vi "MTS_AutoLaserPower.vi"(11 "Laser Color":enum16{"Blue", "Green", "Red"}(ring)) -> (0 "Error ?":bool, 1 "Laser 2 Position":dbl, 2 "Laser 1 Position":dbl, 3 "New Positions":u8[](array[numeric]))   [LabVIEW 2011]
panel:
  out "Progress":u8(slide) scale=0.0..100.0
  out "Laser Power":cluster{dbl[], dbl[]}(graph)
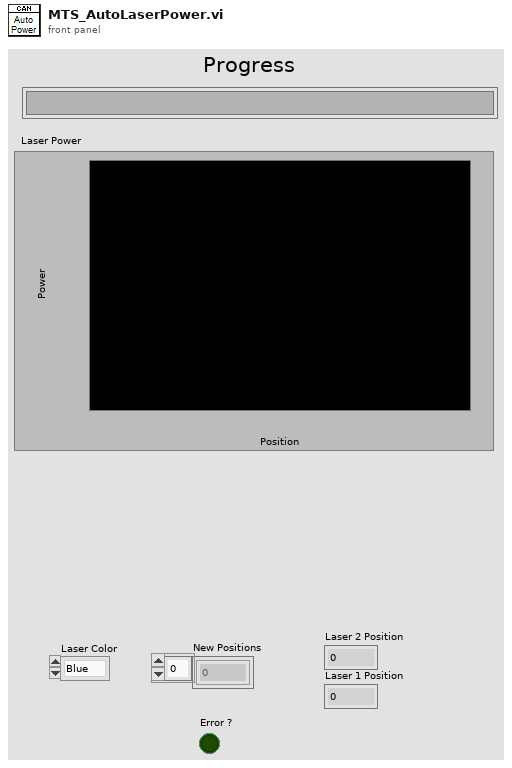
[diagram p1: front panel]
types:
  T1 = enum8{"STD, NO RTR", "STD,RTR", "XTD, NO RTR", "XTD, RTR"}
  T2 = cluster{"x":u32, "MSG type":enum8{"STD, NO RTR", "STD,RTR", "XTD, NO RTR", "XTD, RTR"}, "LEN 3":u8, u8[]}
  T3 = cluster{"x":u32, "MSG type":enum8{"STD, NO RTR", "STD,RTR", "XTD, NO RTR", "XTD, RTR"}, "LEN 3":u8, "Array":u8[]}
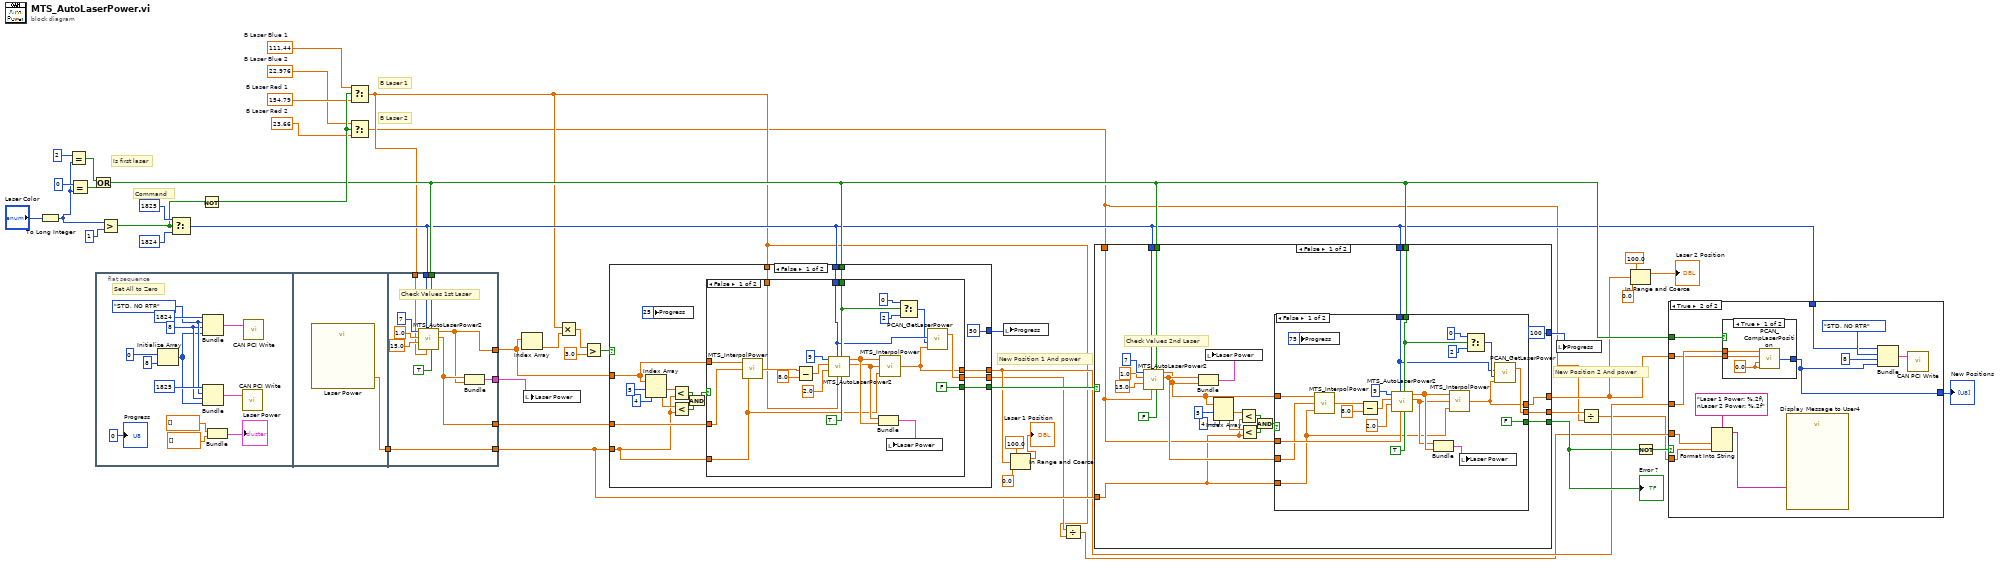
[diagram p0: block diagram]
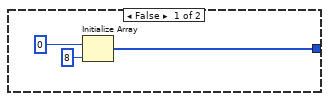
[diagram p2: hidden frame]
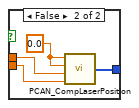
[diagram p3: hidden frame]
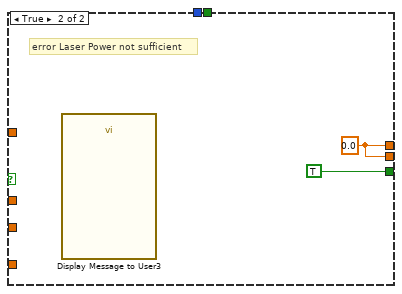
[diagram p4: hidden frame]
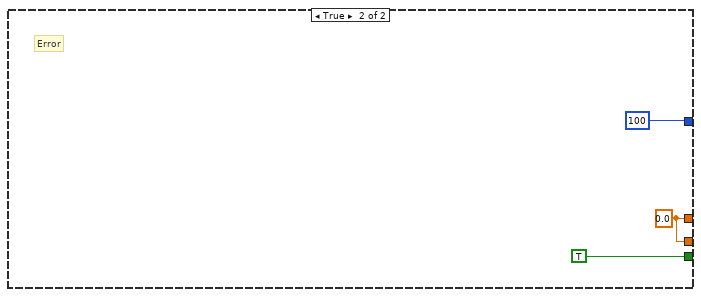
[diagram p5: hidden frame]
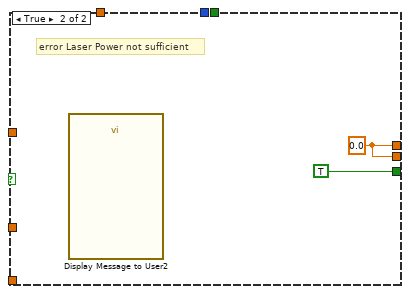
[diagram p6: hidden frame]
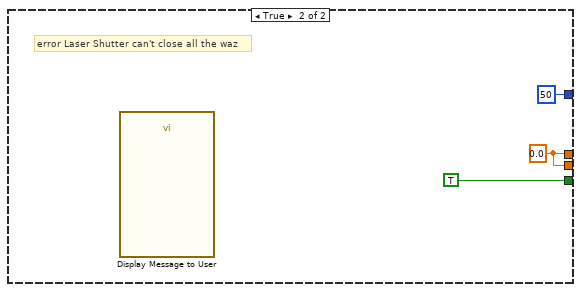
[diagram p7: hidden frame]
diagram:
  w28 = 23.66  # B Laser Red 2
  w30 = 154.79  # B Laser Red 1
  w29 = 22.976  # B Laser Blue 2
  w33 = 111.44  # B Laser Blue 1
  # "New Position 2 And power"
  # "New Position 1 And power"
  # "B Laser 2"
  # "B Laser 1"
  # "Is first laser"
  # "Command"
  n1 = To Long Integer(number="Laser Color") -> (32bit integer=w41:i32)
  n2 = Equal?(x=2, y=w41) -> (x = y?=w38:bool)
  n3 = Equal?(x=0, y=w41) -> (x = y?=w39:bool)
  n4 = Or(x=w38, y=w39) -> (x .or. y?=w21:bool)
  n5 = flat-sequence {
    tunnel: [w60] -> w37
    tunnel: w12 -> [w69]
    tunnel: w21 -> [w70]
    tunnel: [w63] -> w34
    tunnel: [w71] -> w25
    tunnel: w37 -> [w71]
    tunnel: [w64] -> w27
    tunnel: [w62] -> w9
    tunnel: w4 -> [w61]
    frame #0 {
      w54 = T1."STD, NO RTR" ("MSG type")
      w53 = u8 8 ("LEN 3")
      # "Set All to Zero"
      n6 = Initialize Array(u8 0, 8 ("dimension size")) -> (w52:u8[])
      n7 = Bundle("x"=u32 1824, "MSG type"=w54, "LEN 3"=w53, w52) -> (w57:T2)  [unwired: 1 in]
      n8 = Bundle("x"=u32 1825, "MSG type"=w54, "LEN 3"=w53, w52) -> (w51:T2)  [unwired: 1 in]
      n9 = Bundle(dbl[] [], dbl[] []) -> (→"Laser Power":cluster{dbl[], dbl[]})  [unwired: 1 in]
      n10 = call "CAN PCI Write.vi"("CAN_Message"=w51) -> ()  [unwired: 2 in, 1 out]
      n11 = call "CAN PCI Write.vi"("CAN_Message"=w57) -> ()  [unwired: 2 in, 1 out]
      "Progress" <- u8 0 ("Slide")
    }
    frame #1 {
      n12 = call "Laser Power"() -> ("Power ( µW )"=w60:dbl)  [unwired: 17 in, 2 out]
    }
    frame #2 {
      # "Check Values 1st Laser"
      n13 = call "MTS_AutoLaserPower2.vi"("Laser 1/3 ?"=TRUE, "Laser 1-2 ?"=w70, "Laser Power Callib"=w61, "CAN Adress"=w69, "Step"=15.0, "Offset"=1.0, "N Points"=7) -> ("Positions"=w64:dbl[], "Intensitys"=w63:dbl[])  [unwired: 2 in, 1 out]
      n14 = Bundle("Positions"=w64, "Intensitys"=w63) -> (w62:cluster{"Positions":dbl[], "Intensitys":dbl[]})  [unwired: 1 in]
    }
  }
  n15 = Greater?(x=w41, y=1) -> (0:w32:bool)
  n16 = Select(t=u32 1825 ("x"), s=w32, f=u32 1824 ("x")) -> (s? t:f=w12:u32)
  n17 = Not(x=w32) -> (.not. x?=w31:bool)
  n18 = Select(t=w33, s=w31, f=w30) -> (s? t:f=w4:dbl)
  n19 = Select(t=w29, s=w31, f=w28) -> (s? t:f=w1:dbl)
  n20 = Index Array(array=w34) -> (element=w8:dbl)  [unwired: 1 in]
  n21 = local write "Laser Power"(w9) -> ()
  n22 = Multiply(x=w4, y=w8) -> (x*y=w7:dbl)
  n23 = Greater?(x=w7, y=3.0) -> (0:w35:bool)
  n24 = case shown="False" w35 {
    tunnel: w34 -> [w78 _]
    tunnel: w25 -> [w72 _]
    tunnel: [w88 TRUE ("Error ?")] -> w26
    tunnel: w27 -> [w86 _]
    tunnel: w12 -> [w85 _]
    tunnel: w21 -> [w84 _]
    tunnel: [w83 w114] -> w20
    tunnel: [w82 w114] -> w6
    tunnel: [u8 50 ("Slide") u8 50 ("Slide")] -> w11
    tunnel: w4 -> [w79 _]
    frame False {
      n25 = Index Array(array=w78, index #1=5 ("index"), index #2=4 ("index")) -> (element #1=w87:dbl, element #2=w76:dbl)
      n26 = local write "Progress"(u8 25 ("Slide")) -> ()
      n27 = Less?(x=w87, y=w72) -> (x < y?=w75:bool)
      n28 = Less?(x=w76, y=w72) -> (x < y?=w74:bool)
      n29 = And(x=w75, y=w74) -> (x .and. y?=w73:bool)
      n30 = case shown="False" w73 {
        tunnel: [FALSE ("Error ?") TRUE ("Error ?")] -> w88
        tunnel: w78 -> [w110 _]
        tunnel: w86 -> [w109 _]
        tunnel: w72 -> [w91 _]
        tunnel: w85 -> [w96 _]
        tunnel: w84 -> [w98 _]
        tunnel: [w90 w111] -> w83
        tunnel: [w94 w111] -> w82
        tunnel: w79 -> [w100 _]
        frame False {
          n31 = call "MTS_InterpolPower.vi"("Desired Power ( µW )"=w91, "Positions"=w109, "Intensitys"=w110) -> ("Numeric"=w105:dbl)
          n32 = Subtract(x=w105, y=8.0) -> (x-y=w107:dbl)
          n33 = call "MTS_AutoLaserPower2.vi"("Laser 1/3 ?"=TRUE, "Laser 1-2 ?"=w98, "Laser Power Callib"=w100, "CAN Adress"=w96, "Step"=2.0, "Offset"=w107, "N Points"=9) -> ("Positions"=w92:dbl[], "Intensitys"=w93:dbl[])  [unwired: 2 in, 1 out]
          n34 = Bundle("Positions"=w92, "Intensitys"=w93) -> (w101:cluster{"Positions":dbl[], "Intensitys":dbl[]})  [unwired: 1 in]
          n35 = call "MTS_InterpolPower.vi"("Desired Power ( µW )"=w91, "Positions"=w92, "Intensitys"=w93) -> ("Numeric"=w90:dbl)
          n36 = local write "Laser Power"(w101) -> ()
          n37 = Select(t=i16 0 ("Laser No"), s=w98, f=i16 2 ("Laser No")) -> (s? t:f=w95:i16)
          n38 = call "PCAN_GetLaserPower.vi"("Position"=w90, "Laser No"=w95, "CAN Adress"=w96) -> ("Intensity (a.u.)"=w94:dbl)  [unwired: 1 in, 1 out]
        }
        frame True {
          w111 = 0.0 ("Numeric")
          # "error Laser Power not sufficient"
          n39 = call "Display Message to User2"() -> ()  [unwired: 10 in, 2 out]
        }
      }
    }
    frame True {
      w114 = 0.0 ("Numeric")
      # "error Laser Shutter can't close all the waz"
      n40 = call "Display Message to User"() -> ()  [unwired: 10 in, 2 out]
    }
  }
  n41 = local write "Progress"(w11) -> ()
  n42 = In Range and Coerce(upper limit=100.0, x=w20, lower limit=0.0) -> (coerced(x)=→"Laser 1 Position":dbl)  [unwired: 1 out]
  n43 = Divide(x=w6, y=w4) -> (x/y=w5:dbl)
  n44 = case shown="False" w26 {
    tunnel: [w133 TRUE ("Error ?")] -> w24
    tunnel: w21 -> [w135 _]
    tunnel: w12 -> [w134 _]
    tunnel: w25 -> [w116 _]
    tunnel: w1 -> [w118 _]
    tunnel: w21 -> [w132 _]
    tunnel: w12 -> [w131 _]
    tunnel: [w130 w165] -> w14
    tunnel: [w129 w165] -> w3
    tunnel: [u8 100 ("Slide") u8 100 ("Slide")] -> w10
    frame False {
      # "Check Values 2nd Laser"
      n45 = call "MTS_AutoLaserPower2.vi"("Laser 1/3 ?"=FALSE, "Laser 1-2 ?"=w135, "Laser Power Callib"=w118, "CAN Adress"=w134, "Step"=15.0, "Offset"=1.0, "N Points"=7) -> ("Positions"=w127:dbl[], "Intensitys"=w117:dbl[])  [unwired: 2 in, 1 out]
      n46 = Bundle("Positions"=w127, "Intensitys"=w117) -> (w126:cluster{"Positions":dbl[], "Intensitys":dbl[]})  [unwired: 1 in]
      n47 = local write "Laser Power"(w126) -> ()
      n48 = Index Array(array=w117, index #1=5 ("index"), index #2=4 ("index")) -> (element #1=w124:dbl, element #2=w122:dbl)
      n49 = Less?(x=w124, y=w116) -> (x < y?=w121:bool)
      n50 = Less?(x=w122, y=w116) -> (x < y?=w120:bool)
      n51 = And(x=w121, y=w120) -> (x .and. y?=w119:bool)
      n52 = case shown="False" w119 {
        tunnel: [FALSE ("Error ?") TRUE ("Error ?")] -> w133
        tunnel: w117 -> [w146 _]
        tunnel: w127 -> [w145 _]
        tunnel: w131 -> [w148 _]
        tunnel: w132 -> [w149 _]
        tunnel: [w140 w162] -> w130
        tunnel: [w147 w162] -> w129
        tunnel: w118 -> [w153 _]
        tunnel: w116 -> [w141 _]
        frame False {
          n53 = local write "Progress"(u8 75 ("Slide")) -> ()
          n54 = call "MTS_InterpolPower.vi"("Desired Power ( µW )"=w141, "Positions"=w145, "Intensitys"=w146) -> ("Numeric"=w144:dbl)
          n55 = Subtract(x=w144, y=8.0) -> (x-y=w160:dbl)
          n56 = call "MTS_AutoLaserPower2.vi"("Laser 1/3 ?"=TRUE, "Laser 1-2 ?"=w149, "Laser Power Callib"=w153, "CAN Adress"=w148, "Step"=2.0, "Offset"=w160, "N Points"=9) -> ("Positions"=w142:dbl[], "Intensitys"=w143:dbl[])  [unwired: 2 in, 1 out]
          n57 = Bundle("Positions"=w142, "Intensitys"=w143) -> (w154:cluster{"Positions":dbl[], "Intensitys":dbl[]})  [unwired: 1 in]
          n58 = call "MTS_InterpolPower.vi"("Desired Power ( µW )"=w141, "Positions"=w142, "Intensitys"=w143) -> ("Numeric"=w140:dbl)
          n59 = local write "Laser Power"(w154) -> ()
          n60 = Select(t=i16 0 ("Laser No"), s=w149, f=i16 2 ("Laser No")) -> (s? t:f=w150:i16)
          n61 = call "PCAN_GetLaserPower.vi"("Position"=w140, "Laser No"=w150, "CAN Adress"=w148) -> ("Intensity (a.u.)"=w147:dbl)  [unwired: 1 in, 1 out]
        }
        frame True {
          w162 = 0.0 ("Numeric")
          # "error Laser Power not sufficient"
          n62 = call "Display Message to User3"() -> ()  [unwired: 10 in, 2 out]
        }
      }
    }
    frame True {
      w165 = 0.0 ("Numeric")
      # "Error"
    }
  }
  "Error ?" <- w24
  n63 = local write "Progress"(w10) -> ()
  n64 = Divide(x=w3, y=w1) -> (x/y=w2:dbl)
  n65 = In Range and Coerce(upper limit=100.0, x=w14, lower limit=0.0) -> (coerced(x)=→"Laser 2 Position":dbl)  [unwired: 1 out]
  n66 = Not(x=w24) -> (.not. x?=w23:bool)
  n67 = case shown="True" w23 {
    tunnel: w5 -> [_ w180]
    tunnel: w2 -> [_ w179]
    tunnel: [w167 w171] -> w22
    tunnel: w21 -> [_ w177]
    tunnel: w20 -> [_ w176]
    tunnel: w14 -> [_ w175]
    tunnel: w12 -> [_ w170]
    frame False {
      n68 = Initialize Array(u8 0, 8 ("dimension size")) -> (w167:u8[])
    }
    frame True {
      n69 = Format Into String(format string="Laser 1 Power: %.2f\nLaser 2 Power: %.2f", w180, w179) -> (resulting string=w178:string)  [unwired: 2 in, 1 out]
      n70 = case shown="True" w177 {
        tunnel: [w185 w189] -> w171
        tunnel: w176 -> [w184 w186]
        tunnel: w175 -> [w183 w187]
        frame True {
          w182 = 0.0 ("Laser 4")
          n71 = call "PCAN_CompLaserPosition.vi"("Laser 4"=w182, "Laser 3"=w182, "Laser 2"=w183, "Laser 1"=w184) -> ("Array"=w185:u8[])
        }
        frame False {
          w188 = 0.0 ("Laser 4")
          n72 = call "PCAN_CompLaserPosition.vi"("Laser 4"=w187, "Laser 3"=w186, "Laser 2"=w188, "Laser 1"=w188) -> ("Array"=w189:u8[])
        }
      }
      n73 = call "Display Message to User4"("Message"=w178) -> ()  [unwired: 9 in, 2 out]
      n74 = Bundle("x"=w170, "MSG type"=T1."STD, NO RTR", "LEN 3"=u8 8, "Array"=w171) -> (w174:T3)  [unwired: 1 in]
      n75 = call "CAN PCI Write.vi"("CAN_Message"=w174) -> ()  [unwired: 2 in, 1 out]
    }
  }
  "New Positions" <- w22
